vi "Read Flex Ext Wrist.vi"(6 "Error In":errorcluster, 7 "Flex Extension threshold":sgl=55.0, 9 "Leap Handle In":T1) -> (0 "Error Out":errorcluster, 1 "Wrist Flextion/Extension":string="Undetected", 3 "Leap Handle Out":T1)   [LabVIEW 2014]
doc: "<b>Leap Read</b> requests and parses a <b>Frame</b> of data from the Leap Motion Controller. All the data associated with the Frame is organized into a LabVIEW cluster for accessibility.\n\nSpecifics about the data in the Frame cluster can be found by going to <b>Help » Leap Motion Controller Help</b> inside of LabVIEW"
uses:
  Typedef 2.0/Leap Handle.ctl
  C:/Users/Andrea/Desktop/Programmi LabView/Smart Wristband/Smart Wristband/Leap Motion VIs 2.0/LeapCSharp.NET4.0.dll
  LeapCSharp.NET4.0.dll
panel:
  out "Dot Product":sgl
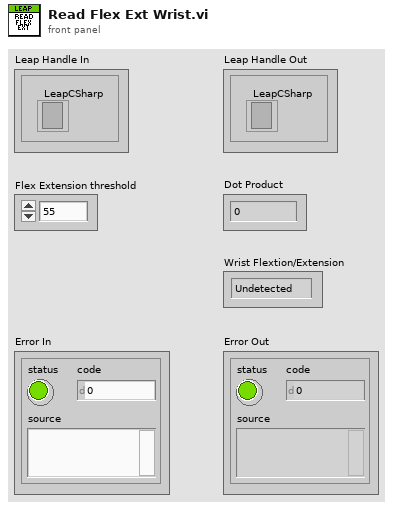
[diagram p1: front panel]
types:
  T1 = typedef "Leap Handle.ctl" = cluster{"LeapCSharp":refnum<k24>}
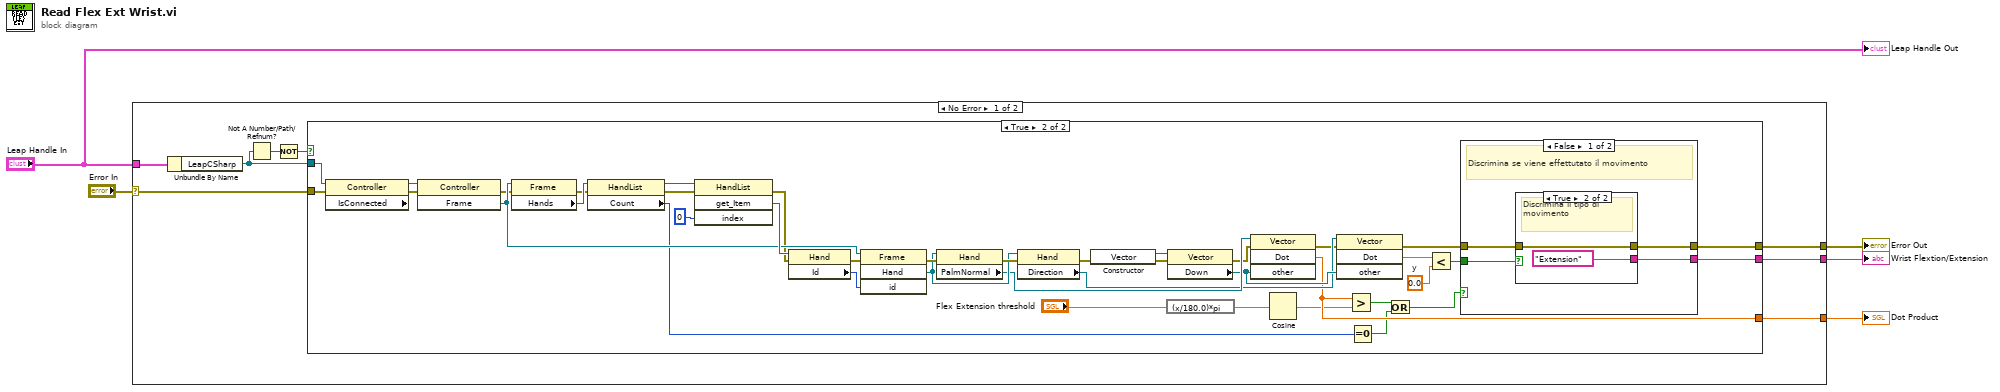
[diagram p0: block diagram]
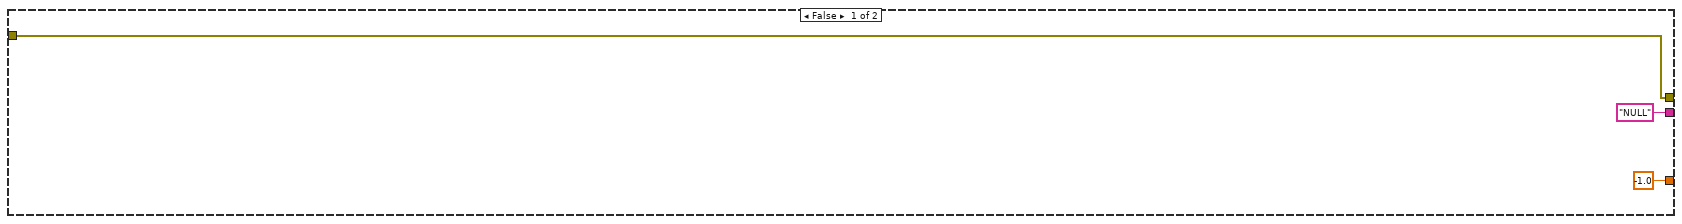
[diagram p2: hidden frame]
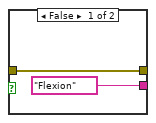
[diagram p3: hidden frame]
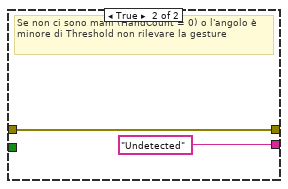
[diagram p4: hidden frame]
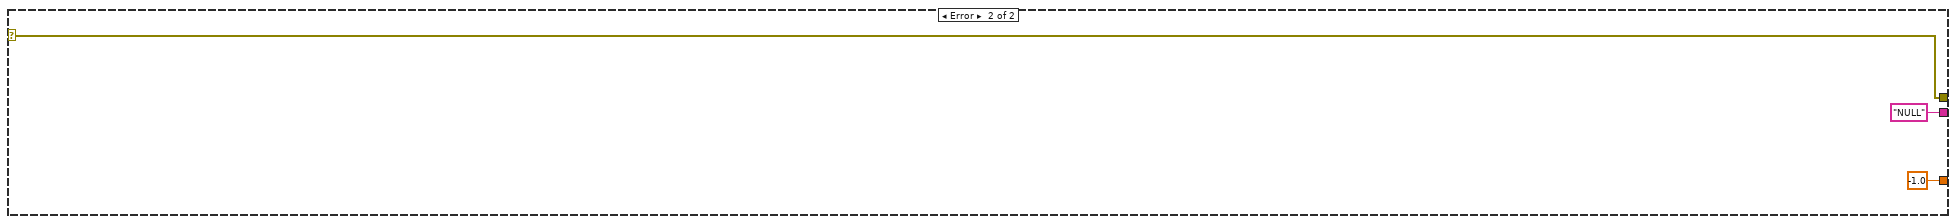
[diagram p5: hidden frame]
diagram:
  n1 = case shown="No Error" "Error In" {
    selector: "Error In" -> [w12 w69]
    tunnel: "Leap Handle In" -> [w13 _]
    tunnel: [w7 w69] -> w4
    tunnel: [w6 sgl -1.0 ("GrabStrength")] -> w3
    tunnel: [w8 "NULL"] -> w1
    frame No Error {
      n2 = Unbundle By Name(w13) -> ("LeapCSharp"=w9:refnum<k24>)
      n3 = Not A Number/Path/Refnum?(number/path/refnum=w9) -> (NaN/Path/Refnum?=w11:bool)
      n4 = Not(x=w11) -> (.not. x?=w10:bool)
      n5 = case shown="True" w10 {
        tunnel: w12 -> [w15 w56]
        tunnel: w9 -> [_ w53]
        tunnel: [sgl -1.0 ("GrabStrength") w24] -> w6
        tunnel: ["NULL" w27] -> w8
        tunnel: [w15 w25] -> w7
        frame False {
        }
        frame True {
          w30 = sgl 0.0  # y
          n6 = property class="Controller" props=["IsConnected"](reference=w53, error in=w56) -> (reference out=w55:refnum<k24>, error out=w54:errorcluster)  [unwired: 1 out]
          n7 = invoke class="Controller" method="Frame"(reference=w55, error in=w54) -> (error out=w46:errorcluster, "Frame"=w47:refnum<k24>)  [unwired: 1 in, 1 out]
          n8 = property class="Frame"(reference=w47, error in=w46) -> (error out=w45:errorcluster, "Hands"=w52:refnum<k24>)  [unwired: 1 out]
          n9 = property class="HandList"(reference=w52, error in=w45) -> (reference out=w51:refnum<k24>, error out=w44:errorcluster, "Count"=w18:i32)
          n10 = invoke class="HandList" method="get_Item"(reference=w51, error in=w44, "index"=0) -> (error out=w43:errorcluster, "get_Item"=w49:refnum<k24>)  [unwired: 1 in, 2 out]
          n11 = property class="Hand"(reference=w49, error in=w43) -> (error out=w42:errorcluster, "Id"=w48:i32)  [unwired: 1 out]
          n12 = invoke class="Frame" method="Hand"(reference=w47, error in=w42, "id"=w48) -> (error out=w41:errorcluster, "Hand"=w37:refnum<k24>)  [unwired: 1 in, 2 out]
          n13 = property class="Hand"(reference=w37, error in=w41) -> (error out=w38:errorcluster, "PalmNormal"=w35:refnum<k24>)  [unwired: 1 out]
          n14 = property class="Hand"(reference=w37, error in=w38) -> (error out=w36:errorcluster, "Direction"=w33:refnum<k24>)  [unwired: 1 out]
          n15 = constructor class="Vector"(error in=w36) -> (reference out=w40:refnum<k24>, error out=w39:errorcluster)  [unwired: 2 in, 1 out]
          n16 = expression code="(x/180.0)*pi" ("degrees to radians")("Flex Extension threshold") -> (w23:sgl)
          n17 = property class="Vector"(reference=w40, error in=w39) -> (error out=w32:errorcluster, "Down"=w34:refnum<k24>)  [unwired: 1 out]
          n18 = invoke class="Vector" method="Dot"(reference=w35, error in=w32, "other"=w34) -> (error out=w31:errorcluster, "Dot"=w24:sgl)  [unwired: 1 in, 2 out]
          n19 = Cosine(x=w23) -> (cos(x)=w21:sgl)
          n20 = invoke class="Vector" method="Dot"(reference=w33, error in=w31, "other"=w34) -> (error out=w26:errorcluster, "Dot"=w29:sgl)  [unwired: 1 in, 2 out]
          n21 = Greater?(x=w24, y=w21) -> (0:w20:bool)
          n22 = Equal To 0?(x=w18) -> (x = 0?=w17:bool)
          n23 = Or(x=w20, y=w17) -> (x .or. y?=w19:bool)
          n24 = Less?(x=w29, y=w30) -> (x < y?=w28:bool)
          n25 = case shown="False" w19 {
            tunnel: w28 -> [w60 _]
            tunnel: [w59 "Undetected"] -> w27
            tunnel: w26 -> [w58 w66]
            tunnel: [w57 w66] -> w25
            frame False {
              # "Discrimina se viene effettutato il movimento"
              n26 = case shown="True" w60 {
                tunnel: ["Flexion" "Extension"] -> w59
                tunnel: w58 -> [w61 w63]
                tunnel: [w61 w63] -> w57
                frame False {
                }
                frame True {
                  # "Discrimina il tipo di movimento"
                }
              }
            }
            frame True {
              # "Se non ci sono mani (HandCount = 0) o l'angolo è minore di Threshold non rilevare la gesture"
            }
          }
        }
      }
    }
    frame Error {
    }
  }
  "Error Out" <- w4
  "Dot Product" <- w3
  "Wrist Flextion/Extension" <- w1
  "Leap Handle Out" <- "Leap Handle In"
